vi "threshold_manager.vi"() -> ()   [LabVIEW 2018]
uses:
  <vilib>/rvi/DataTransferAndStorage/Container/XNode/niFpgaContainer.xnode
  <vilib>/rvi/Memory/Memory_Emulation/nirvimemoryFastEmulation.vi
  <vilib>/rvi/Memory/Memory_Emulation/nirvimemoryEmulation.vi
panel:
  in  "Numeric":u8
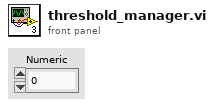
[diagram p1: front panel]
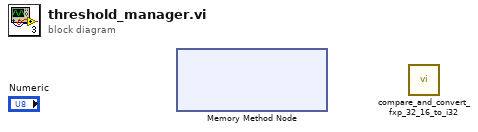
[diagram p0: block diagram]
diagram:
  n1 = xnode ("Memory Method Node")() -> ()  [unwired: 2 in, 2 out]
  n2 = call "compare_and_convert_fxp_32_16_to_i32.vi"() -> ()  [unwired: 3 in, 2 out]
